vi "move step size.vi"(10 "Velocity value (units/s) in":dbl, 11 "Displacement (units)":dbl) -> (0 "error out":errorcluster, 3 "Current position (units)":dbl)   [LabVIEW 2011]
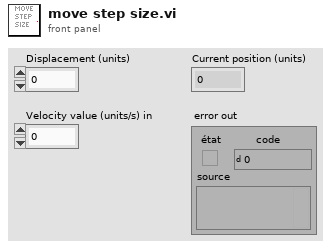
[diagram p1: front panel]
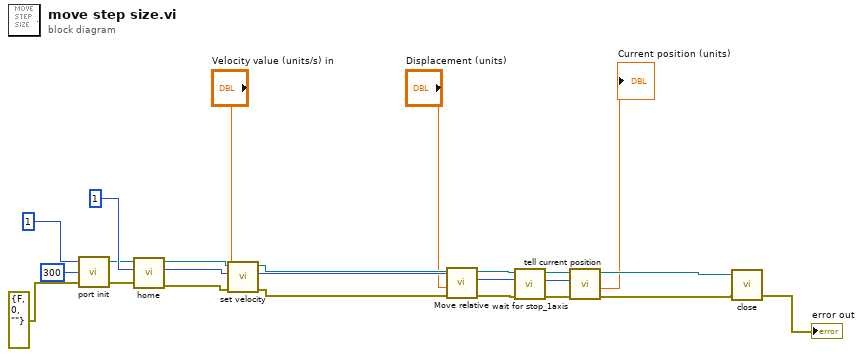
[diagram p0: block diagram]
diagram:
  n1 = call <userlib>:"port init.vi"("error in"=errorcluster {"status"=FALSE, "code"=0, "source"=""}, "Timeout (ms)"=u32 300, "SerialPort"=u8 1) -> ("error out"=w5:errorcluster, "Visa Handle"=w4:refnum<visa-resource-name>)  [unwired: 1 in]
  n2 = call <userlib>:"home.vi"("error in"=w5, "Axis in"=1, "VISA Handle in"=w4) -> ("error out"=w15:errorcluster, "Axis out"=w13:i32, "VISA Handle out"=w12:refnum<visa-resource-name>)  [unwired: 3 in, 1 out]
  n3 = call <userlib>:"set velocity.vi"("error in"=w15, "Velocity value (units/s)"="Velocity value (units/s) in", "Axis in"=w13, "VISA Handle in"=w12) -> ("error out"=w18:errorcluster, "Axis out"=w19:i32, "VISA Handle out"=w17:refnum<visa-resource-name>)  [unwired: 2 in, 1 out]
  n4 = call <userlib>:"Move relative.vi"("error in"=w18, "Displacement (units)"="Displacement (units)", "Axis in"=w19, "VISA Handle in"=w17) -> ("error out"=w22:errorcluster, "Axis out"=w21:i32, "VISA Handle out"=w20:refnum<visa-resource-name>)  [unwired: 2 in, 1 out]
  n5 = call <userlib>:"wait for stop_1axis.vi"("error in"=w22, "Axis in"=w21, "VISA Handle in"=w20) -> ("error out"=w9:errorcluster, "Axis out"=w8:i32, "VISA Handle out"=w7:refnum<visa-resource-name>)  [unwired: 3 in, 1 out]
  n6 = call <userlib>:"tell current position.vi"("error in"=w9, "Axis in"=w8, "VISA Handle in"=w7) -> ("error out"=w24:errorcluster, "Current position (units)"=→"Current position (units)":dbl, "VISA Handle out"=w23:refnum<visa-resource-name>)  [unwired: 2 in, 2 out]
  n7 = call <userlib>:"close.vi"("error in"=w24, "VISA Handle in"=w23) -> ("error out"=→"error out":errorcluster)  [unwired: 3 in]
